vi "Read Loop.vi"(7 "Enum - Menu":enum16{"INIT", "READ", "RE-INIT", "CLOSE"}(ring), 8 "error in (no error)":errorcluster) -> (0 "error out":errorcluster, 1 "Isolated Gain":u32, 2 "DAQ Status":u32, 3 "Downlink Packet":T1, 4 "rx command count":u32, 5 "Current Filter Id":u32, 6 "Last Config Rejected":u32)   [LabVIEW 2025]
panel:
  out "data out":string
  out "error out 2":errorcluster
  out "connection ID":refnum<k16>
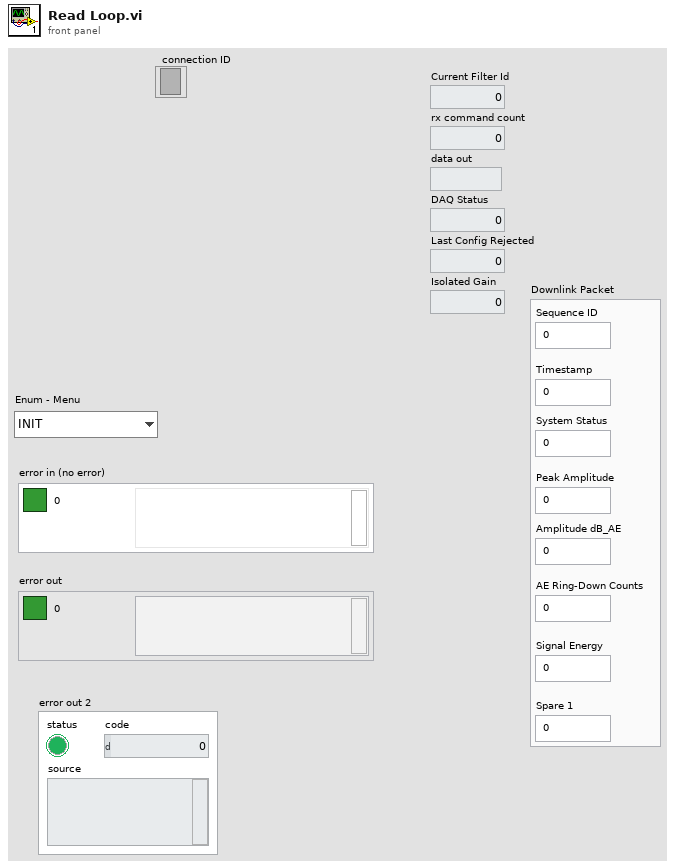
[diagram p1: front panel]
types:
  T1 = cluster{"Sequence ID":u32, "Timestamp":u32, "System Status":u32, "Peak Amplitude":u32, "Amplitude dB_AE":u32, "AE Ring-Down Counts":u32, "Signal Energy":u32, "Spare 1":u32}
  T2 = cluster{"Sequence ID":u32, "Timestamp":u32, "System Status":u32, "Peak Amplitude":sgl, "Amplitude dB_AE":sgl, "AE Ring-Down Counts":u32, "Signal Energy":sgl, "Spare 1":u32}
  T3 = enum16{"big-endian, network order", "native, host order", "little-endian"}
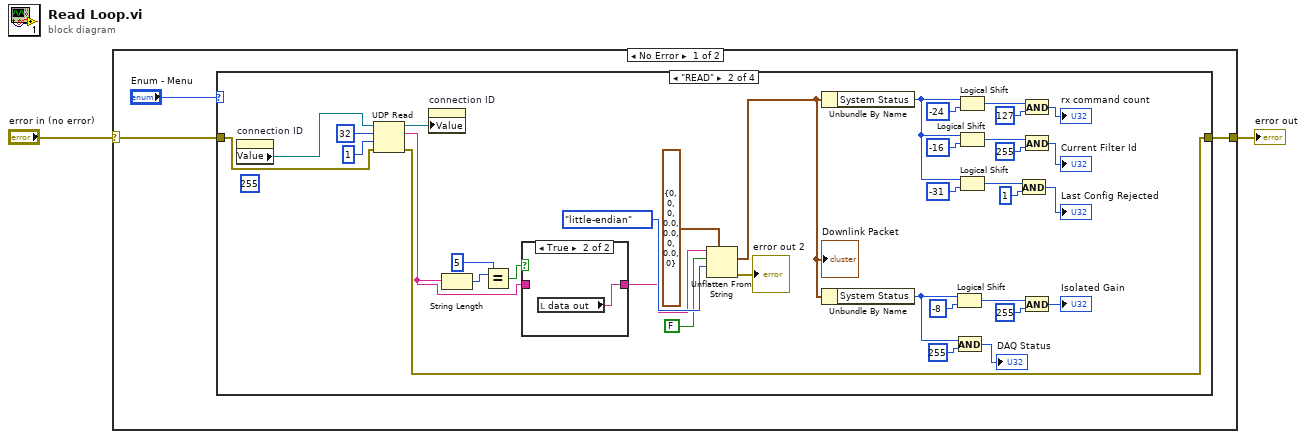
[diagram p0: block diagram]
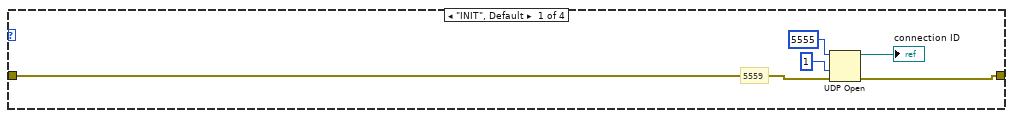
[diagram p2: hidden frame]
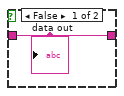
[diagram p3: hidden frame]
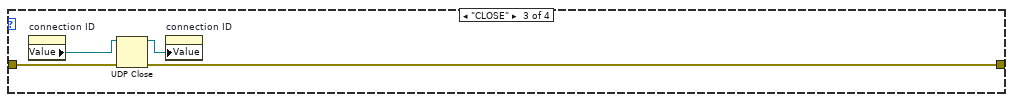
[diagram p4: hidden frame]
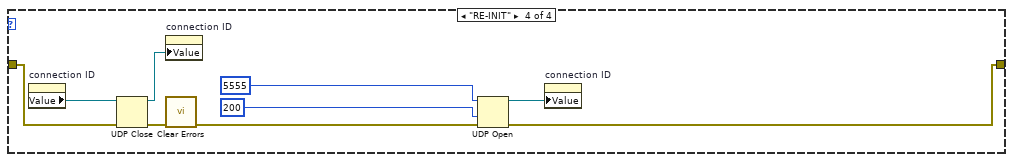
[diagram p5: hidden frame]
diagram:
  n1 = case shown="No Error" "error in (no error)" {
    selector: "error in (no error)" -> [w4 _]
    tunnel: [w3 _] -> w1
    frame No Error {
      n2 = case shown="\"READ\"" "Enum - Menu" {
        tunnel: w4 -> [w9 w46 w50 w61]
        tunnel: [w8 w45 w49 w56] -> w3
        frame "INIT", Default {
          # "5559"
          n3 = UDP Open(8:w9, 9:1 ("timeout ms (25000)"), 11:u16 5555 ("port")) -> (port=→"connection ID":refnum<k16>, 0:w8:errorcluster)  [unwired: 2 in, 1 out]
        }
        frame "READ" {
          (unwired) u32 255
          n4 = property on="connection ID" class="Ref (strict)"() -> ("Value"=w43:refnum<k16>)  [unwired: 2 in, 2 out]
          n5 = UDP Read(connection ID=w43, max size (548)=32, timeout ms (25000)=1, 8:w46) -> (data out=w12:string, error out=w45:errorcluster, 3:w44:refnum<k16>)  [unwired: 2 out]
          n6 = property on="connection ID" class="Ref (strict)"("Value"=w44) -> ()  [unwired: 2 in, 2 out]
          n7 = String Length(string=w12) -> (length=w15:i32)
          n8 = Equal?(x=w15, y=5) -> (x = y?=w13:bool)
          n9 = case shown="True" w13 {
            tunnel: w12 -> [w47 _]
            tunnel: [w47 w48] -> w11
            frame False {
              "data out" <- w47
            }
            frame True {
              n10 = local read "data out"() -> (w48:string)
            }
          }
          n11 = Unflatten From String(type=T2 {"Sequence ID"=0, "Timestamp"=0, "System Status"=0, "Peak Amplitude"=0.0, "Amplitude dB_AE"=0.0, "AE Ring-Down Counts"=0, "Signal Energy"=0.0, "Spare 1"=0} ("Downlink Packet"), binary string=w11, data includes array or string size? (T)=FALSE ("prepend array or string size? (T)"), byte order (0:big-endian, network order)=T3."little-endian") -> (value=w29:T2, error out=→"error out 2":errorcluster)  [unwired: 1 in, 1 out]
          "Downlink Packet" <- w29
          n12 = Unbundle By Name(w29) -> ("System Status"=w16:u32)
          n13 = Unbundle By Name(w29) -> ("System Status"=w35:u32)
          n14 = Logical Shift(y=w35, x=-8) -> (x << y=w33:i32)
          n15 = And(x=w35, y=u32 255) -> (x .and. y?=→"DAQ Status":u32)
          n16 = Logical Shift(y=w16, x=-24) -> (x << y=w22:i32)
          n17 = Logical Shift(y=w16, x=-16) -> (x << y=w27:i32)
          n18 = Logical Shift(y=w16, x=-31) -> (x << y=w19:i32)
          n19 = And(x=w19, y=u32 1) -> (x .and. y?=→"Last Config Rejected":u32)
          n20 = And(x=w22, y=u32 127) -> (x .and. y?=→"rx command count":u32)
          n21 = And(x=w27, y=u32 255) -> (x .and. y?=→"Current Filter Id":u32)
          n22 = And(x=w33, y=u32 255) -> (x .and. y?=→"Isolated Gain":u32)
        }
        frame "CLOSE" {
          n23 = property on="connection ID" class="Ref (strict)"() -> ("Value"=w52:refnum<k16>)  [unwired: 2 in, 2 out]
          n24 = UDP Close(connection ID=w52, 8:w50) -> (connection ID out=w51:refnum<k16>, error out=w49:errorcluster)
          n25 = property on="connection ID" class="Ref (strict)"("Value"=w51) -> ()  [unwired: 2 in, 2 out]
        }
        frame "RE-INIT" {
          n26 = property on="connection ID" class="Ref (strict)"() -> ("Value"=w60:refnum<k16>)  [unwired: 2 in, 2 out]
          n27 = UDP Close(connection ID=w60, 8:w61) -> (connection ID out=w59:refnum<k16>, error out=w57:errorcluster)
          n28 = property on="connection ID" class="Ref (strict)"("Value"=w59) -> ()  [unwired: 2 in, 2 out]
          n29 = call <vilib>:"Clear Errors.vi"("error in (no error)"=w57) -> ("error out"=w54:errorcluster)  [unwired: 5 in, 1 out]
          n30 = UDP Open(8:w54, 9:200 ("timeout ms (25000)"), 11:u16 5555 ("port")) -> (port=w55:refnum<k16>, 0:w56:errorcluster)  [unwired: 2 in, 1 out]
          n31 = property on="connection ID" class="Ref (strict)"("Value"=w55) -> ()  [unwired: 2 in, 2 out]
        }
      }
    }
    frame Error {
    }
  }
  "error out" <- w1
